vi "Hitrap_DiagnosticBoxGUI.checkPositionReached.vi"(0 "referenced?":bool=TRUE, 1 "actPosition []":dbl, 2 "desired Position":dbl, 4 "wrong steps":i32=1) -> (16 "Position Reached?":bool)   [LabVIEW 2014, in "Hitrap_DiagnosticBoxGUI.lvlib"]
doc: "indicates whether the desired position is reached"
uses:
  Hitrap_DiagnosticBoxGUI.lvlib
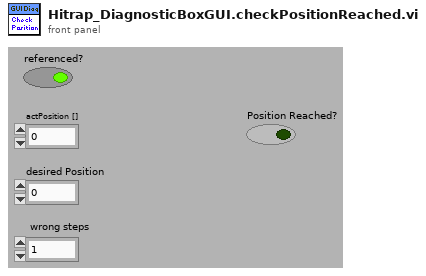
[diagram p1: front panel]
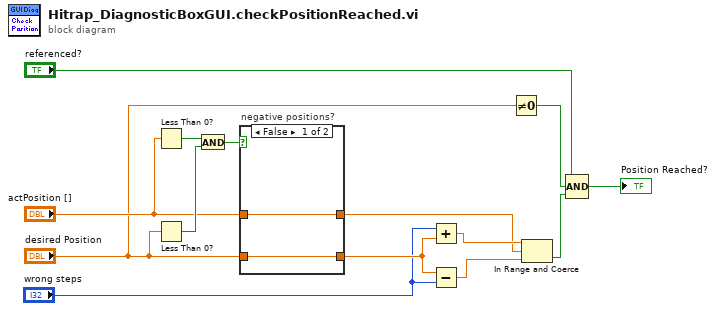
[diagram p0: block diagram]
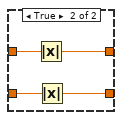
[diagram p2: hidden frame]
diagram:
  n1 = Less Than 0?(x="actPosition []") -> (x < 0?=w12:bool)
  n2 = Less Than 0?(x="desired Position") -> (x < 0?=w11:bool)
  n3 = And(x=w12, y=w11) -> (x .and. y?=w10:bool)
  n4 = case "negative positions?" shown="False" w10 {
    tunnel: "actPosition []" -> [w16 w20]
    tunnel: [w16 w19] -> w8
    tunnel: "desired Position" -> [w15 w18]
    tunnel: [w15 w17] -> w7
    frame False {
    }
    frame True {
      n5 = Absolute Value(x=w20) -> (abs(x)=w19:dbl)
      n6 = Absolute Value(x=w18) -> (abs(x)=w17:dbl)
    }
  }
  n7 = Add(x="wrong steps", y=w7) -> (x+y=w14:dbl)
  n8 = Subtract(x=w7, y="wrong steps") -> (x-y=w13:dbl)
  n9 = Not Equal To 0?(x="desired Position") -> (x != 0?=w3:bool)
  n10 = In Range and Coerce(upper limit=w14, x=w8, lower limit=w13) -> (In Range?=w4:bool)  [unwired: 1 out]
  n11 = Compound Arithmetic op=AND("referenced?", w3, w4) -> (→"Position Reached?":bool)
